vi "SCCSup LineStringToArray.vi"(1 "delimiter (Tab)":string, 2 "line string":string, 4 "remove last empty element? (T)":bool=TRUE) -> (7 "line array":string[](array[string]))   [LabVIEW 2017]
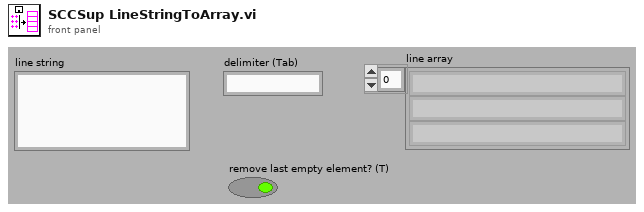
[diagram p1: front panel]
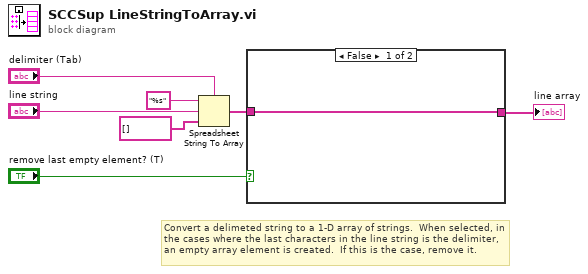
[diagram p0: block diagram]
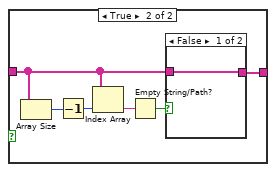
[diagram p2: hidden frame]
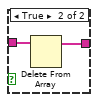
[diagram p3: hidden frame]
diagram:
  # "Convert a delimeted string to a 1-D array of strings.  When selected, in the cases where the last characters in the line string is the delimiter, an empty array element is created.  If this is the case, remove it."
  n1 = Spreadsheet String To Array(delimiter (Tab)="delimiter (Tab)", format string="%s", spreadsheet string="line string", array type (2D Dbl)=string[] []) -> (array=w3:string[])
  n2 = case shown="False" "remove last empty element? (T)" {
    tunnel: w3 -> [w8 w12]
    tunnel: [w8 w9] -> w2
    frame False {
    }
    frame True {
      n3 = Array Size(array=w12) -> (size(s)=w14:i32)
      n4 = Decrement(x=w14) -> (x-1=w13:i32)
      n5 = Index Array(array=w12, index=w13) -> (element=w11:string)
      n6 = Empty String/Path?(string/path=w11) -> (empty?=w10:bool)
      n7 = case shown="False" w10 {
        tunnel: w12 -> [w15 w17]
        tunnel: [w15 w16] -> w9
        frame False {
        }
        frame True {
          n8 = Delete From Array(array=w17) -> (array with subset deleted=w16:string[])  [unwired: 2 in, 1 out]
        }
      }
    }
  }
  "line array" <- w2
